vi "centered_ring_bounds.vi"(5 "radius R":dbl) -> (1 "Bounding Rectangle":T1)   [LabVIEW 2011]
doc: "Creates a bounding rectangle for a overlay ring of radius R centerd in the image."
uses:
  global_vars.vi
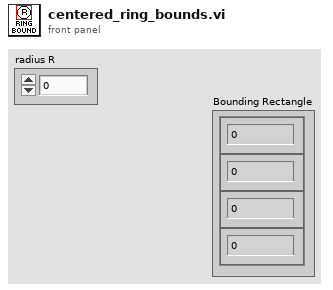
[diagram p1: front panel]
types:
  T1 = cluster{"Numeric Control":dbl, "Numeric Control":dbl, "Numeric Control":dbl, "Numeric Control":dbl}
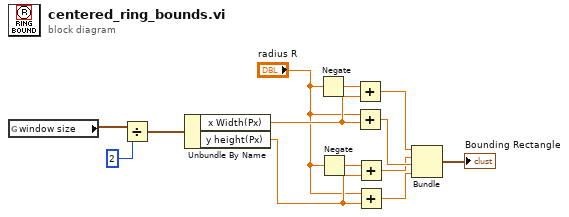
[diagram p0: block diagram]
diagram:
  n1 = global read "global_vars.vi" "window size"() -> (w2:cluster{"x Width(Px)":i32, "y height(Px)":i32})
  n2 = Divide(x=w2, y=2 ("y height(Px)")) -> (x/y=w1:cluster{"x Width(Px)":dbl, "y height(Px)":dbl})
  n3 = Unbundle By Name(w1) -> ("x Width(Px)"=w11:dbl, "y height(Px)"=w7:dbl)
  n4 = Negate(x="radius R") -> (-x=w12:dbl)
  n5 = Negate(x="radius R") -> (-x=w8:dbl)
  n6 = Add(x=w12, y=w11) -> (x+y=w10:dbl)
  n7 = Add(x="radius R", y=w11) -> (x+y=w9:dbl)
  n8 = Add(x=w8, y=w7) -> (x+y=w5:dbl)
  n9 = Add(x="radius R", y=w7) -> (x+y=w4:dbl)
  n10 = Bundle(w10, w5, w9, w4) -> (→"Bounding Rectangle":cluster{dbl, dbl, dbl, dbl})  [unwired: 1 in]
